vi "Image_Crop_Fixed.vi"(8 "Particle Measurements":dbl[][](array[numeric])=[[57.0, 126.0, 60.0, 134.0, 14.0], [248.0, 156.0, 341.0, 306.0, 6231.0], [31.0, 193.0, 32.0, 194.0, 1.0], [324.0, 201.0, 327.0, 209.0, 15.0], [350.0, 252.0, 359.0, 273.0, 108.0], [55.0, 573.0, 56.0, 576.0, 3.0]], 9 "Image  in":T1, 11 "Data":T2={"L16 Linear Actuator"="", "XE 1000 Pump"="", "Camera1"="", "Camera2"="", "Camera1_IMG"=refnum, "Camera2_IMG"=refnum, "Img_Capt"=FALSE, "Actuator"=FALSE, "Pump"=FALSE, "Cam 1"=FALSE, "Cam 2"=FALSE, "Empty_Refill"=FALSE, "Crop"=FALSE, "Light intensity"=100, "Exposure Time"=1000.0, "Sample Name"="Test Sample", "Operator"="MRJ", "Calibration 1"=path "C:/Users/au540322/Desktop/IHS_Project/images/Debris/Debris_0/Debris_0_2019_06_01-23-32-49-686.PNG", "Calibration 2"=path "C:/Users/au540322/Desktop/IHS_Project/images/Debris/Debris_0/Debris_0_2019_06_01-23-32-49-686.PNG", "Framerate"=1, "Timeout Sample"=0, "Collection date"="MRJ", "Sample size threshold"=1, "Empty start"=1, "Command"="MRJ", "Calibration Image 1"=refnum, "Calibration Image 2"=refnum, "Original Image 1"=refnum, "Original Image 2"=refnum, "Processing Image 1"=refnum, "Processing Image 2"=refnum, "Object Image 1"=refnum, "Object Image 2"=refnum, "Cam 1 - save queue"=refnum, "Cam 2 - save queue"=refnum, "Station"="", "Species Name"="", "Other Notes"="", "Aperture"=enum."Item 0", "Image Process Queue Size"=500, "Image Save Queue Size"=500, "Overload threshold"=500, "Max Framerate"=100, "Blue Plane Image"=refnum, "Subtract Image"=refnum, "Binary Image 1"=refnum, "ROI mask allocation"=refnum, "Rectangle 1"={"Left"=0, "Top"=0, "Right"=0, "Bottom"=0, "Rotation"=0.0}, "Rectangle 2"={"Left"=0, "Top"=0, "Right"=0, "Bottom"=0, "Rotation"=0.0}, "Binary Image 2"=refnum, "Detection Region %"=0.0, "Cam 1 queue"=refnum, "Cam 2 queue"=refnum, "Detect image 1"=refnum, "Detect image 2"=refnum, "Detect 1"=path "C:/Users/au540322/Desktop/IHS_Project/images/Debris/Debris_0/Debris_0_2019_06_01-23-32-49-686.PNG", "Detect 2"=path "C:/Users/au540322/Desktop/IHS_Project/images/Debris/Debris_0/Debris_0_2019_06_01-23-32-49-686.PNG", "Max large object threshold"=0, "Open(T)/Close(F)"=FALSE} {"Rectangle 2"."Rotation" format="%.2f"; "Rectangle 2"."Left" scale=0.0..1024.0; "Rectangle 2"."Right" scale=0.0..1024.0; "Rectangle 1"."Rotation" format="%.2f"; "Rectangle 1"."Left" scale=0.0..1024.0; "Rectangle 1"."Right" scale=0.0..1024.0; "Max Framerate" min=1; "Overload threshold" min=1; "Image Save Queue Size" min=1; "Image Process Queue Size" min=1; "Empty start" min=1; "Sample size threshold" min=1; "Framerate" min=1; "Light intensity" scale=0.0..100.0}) -> (0 "ROI descriptor":T5={"Global Rectangle"=[233, 141, 356, 321], "Contours"=[{"ID"=enum."External", "Type"=3, "Coordinates"=[233, 141, 356, 321]}]}, 2 "Object accept":bool=TRUE, 3 "Object":bool)   [LabVIEW 2019]
uses:
  controls/Data.ctl
  <vilib>/userdefined/High Color/IMAQdx.ctl
  <vilib>/vision/Image Controls.llb/IMAQ Image.ctl
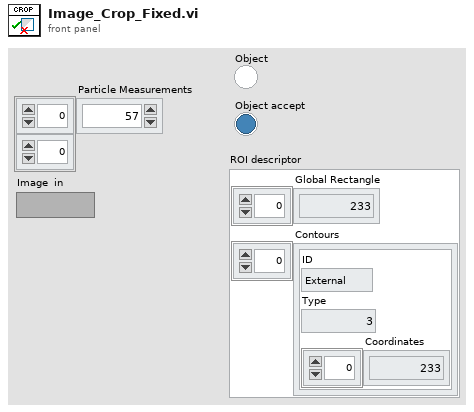
[diagram p1: front panel]
types:
  T1 = typedef "IMAQ Image.ctl" = refnum<image>
  T2 = typedef "Data.ctl" = cluster{"L16 Linear Actuator":refnum<visa-resource-name>, "XE 1000 Pump":refnum<visa-resource-name>, "Camera1":T3, "Camera2":T3, "Camera1_IMG":T1, "Camera2_IMG":T1, "Img_Capt":bool, "Actuator":bool, "Pump":bool, "Cam 1":bool, "Cam 2":bool, "Empty_Refill":bool, "Crop":bool, "Light intensity":i32, "Exposure Time":dbl, "Sample Name":string, "Operator":string, "Calibration 1":path, "Calibration 2":path, "Framerate":i32, "Timeout Sample":i32, "Collection date":string, "Sample size threshold":i32, "Empty start":u32, "Command":string, "Calibration Image 1":T1, "Calibration Image 2":T1, "Original Image 1":T1, "Original Image 2":T1, "Processing Image 1":T1, "Processing Image 2":T1, "Object Image 1":T1, "Object Image 2":T1, "Cam 1 - save queue":refnum<queue>, "Cam 2 - save queue":refnum<queue>, "Station":string, "Species Name":string, "Other Notes":string, "Aperture":enum32{"Item 0", "Item 1", "Item 2", "Item 3"}, "Image Process Queue Size":i32, "Image Save Queue Size":i32, "Overload threshold":i32, "Max Framerate":i32, "Blue Plane Image":T1, "Subtract Image":T1, "Binary Image 1":T1, "ROI mask allocation":T1, "Rectangle 1":T4, "Rectangle 2":T4, "Binary Image 2":T1, "Detection Region %":dbl, "Cam 1 queue":refnum<queue>, "Cam 2 queue":refnum<queue>, "Detect image 1":T1, "Detect image 2":T1, "Detect 1":path, "Detect 2":path, "Max large object threshold":i32, "Open(T)/Close(F)":bool}
  T3 = typedef "IMAQdx.ctl" = refnum<k21>
  T4 = typedef "IMAQ Rectangle" = cluster{"Left":i32, "Top":i32, "Right":i32, "Bottom":i32, "Rotation":dbl}
  T5 = cluster{"Global Rectangle":i32[], "Contours":cluster{"ID":enum32{"External", "Internal"}, "Type":u32, "Coordinates":i32[]}[]}
  T6 = cluster{"ID":enum32{"External", "Internal"}, "Type":u32, "Coordinates":i32[]}[]
  T7 = cluster{"ID":enum32{"External", "Internal"}, "Type":u32, "Coordinates":i32[]}
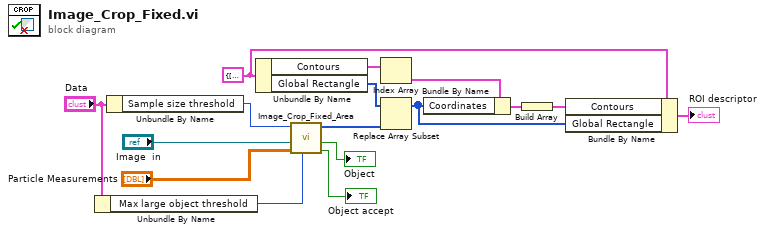
[diagram p0: block diagram]
diagram:
  w9 = T5 {"Global Rectangle"=[106, 29, 356, 265], "Contours"=[{"ID"=enum."External", "Type"=3, "Coordinates"=[106, 29, 356, 265]}]} ("Crop to object")
  n1 = Unbundle By Name("Data") -> ("Max large object threshold"=w1:i32)
  n2 = Unbundle By Name("Data") -> ("Sample size threshold"=w7:i32)
  n3 = Unbundle By Name(w9) -> ("Contours"=w15:T6, "Global Rectangle"=w16:i32[])
  n4 = call "Image_Crop_Fixed_Area.vi"("Large object threshold"=w1, "Particle Measurements in"="Particle Measurements", "Image  in"="Image  in", "Object size threshold"=w7) -> ("Object accept"=→"Object accept":bool, "Object"=→"Object":bool, "Crop coordinates array"=w8:i32[])  [unwired: 5 in]
  n5 = Index Array(array=w15) -> (element=w14:T7)  [unwired: 1 in]
  n6 = Replace Array Subset(array=w16, new element=w8) -> (w13:i32[])  [unwired: 1 in]
  n7 = Bundle By Name(cluster=w14, "Coordinates"=w13) -> (w12:T7)
  n8 = Build Array(w12) -> (w11:T6)
  n9 = Bundle By Name(cluster=w9, "Contours"=w11, "Global Rectangle"=w13) -> (→"ROI descriptor":T5)
